vi "Write Resource.vi"(8 "error in (no error)":errorcluster, 10 "Resource":refnum<visa-resource-name>, 11 "PowerSupplyVisa in":refnum<class "PowerSupplyVisa.lvclass">) -> (0 "error out":errorcluster, 3 "PowerSupplyVisa out":refnum<class "PowerSupplyVisa.lvclass">)   [LabVIEW 2020, in "LAF2024Q2.lvlib" / "PowerSupplyVisa.lvclass"]
uses:
  PowerSupplyVisa.lvclass
  PowerSupplyVisa.lvclass/PowerSupplyVisa.ctl
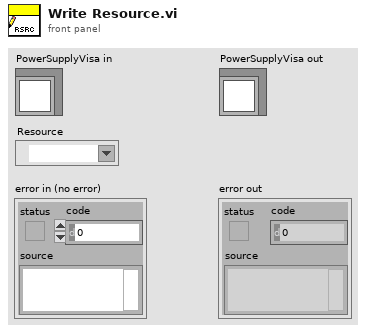
[diagram p1: front panel]
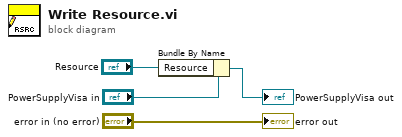
[diagram p0: block diagram]
diagram:
  n1 = Bundle By Name(cluster="PowerSupplyVisa in", "Resource"="Resource") -> (→"PowerSupplyVisa out":refnum<class "PowerSupplyVisa.lvclass">)
  "error out" <- "error in (no error)"
